vi "SetIFGateTrackProp.vi"(8 "错误输入（无错误）":errorcluster, 10 "闸门跟踪属性":u16) -> (0 "错误输出":errorcluster)   [LabVIEW 2014]
uses:
  ZXUTConfigMgr.dll
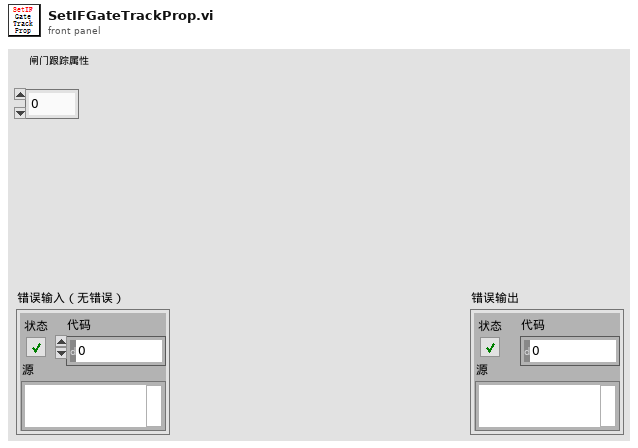
[diagram p1: front panel]
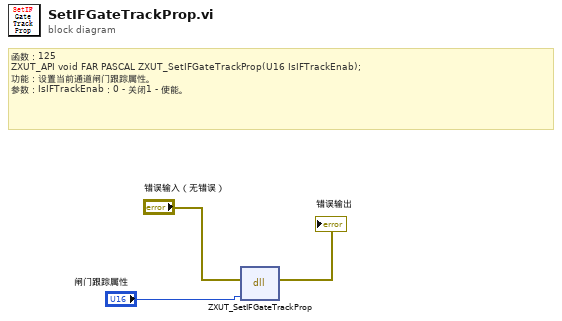
[diagram p0: block diagram]
diagram:
  # "函数：125\nZXUT_API void\tFAR PASCAL ZXUT_SetIFGateTrackProp(U16 IsIFTrackEnab);\n功能：设置当前通道闸门跟踪属性。\n参数：IsIFTrackEnab：0 - 关闭1 - 使能。"
  n1 = dll-call lib="PTH2eabs D软件超声实时监测软件ZXUTAppDemo(华南理工V02.00)X86DllZXUTConfigMgr.dll" fn="ZXUT_SetIFGateTrackProp"(error in="错误输入（无错误）", "IsIFTrackEnab"="闸门跟踪属性") -> (error out=→"错误输出":errorcluster)  [unwired: 4 in, 1 out]
